vi "Result_Test.vi"(8 "error in (no error)":errorcluster caption="entrée d'erreur (pas d'erreur)", 11 "Get_Voltage en entrée":refnum<class "P2056_Get_SN.lvclass">) -> (0 "error out":errorcluster caption="sortie d'erreur", 3 "Get_Voltage en sortie":refnum<class "P2056_Get_SN.lvclass">)   [LabVIEW 2020, in "Library Test.lvlib" / "P2056_Get_SN.lvclass"]
uses:
  P2056_Get_SN.lvclass
  C:/Users/ngarcin/OneDrive - Altyor/Standard TB/Suite TB45/Class/Test/Test (Default)/Test (Default).lvclass
  Commun VI/TypeDef/Variable Printable.ctl
  JSON API/JSON Value/Set from JSON string.vi
  JSON API/JSON Value/JSON Value.lvclass
  P2056_Send_Command_UART.lvclass
  JSON API/Variant JSON/Variant JSON.lvlib
  JSON API/Get Polymorphic/JSON GetSet.lvlib
  Commun VI/Library Commun.lvlib
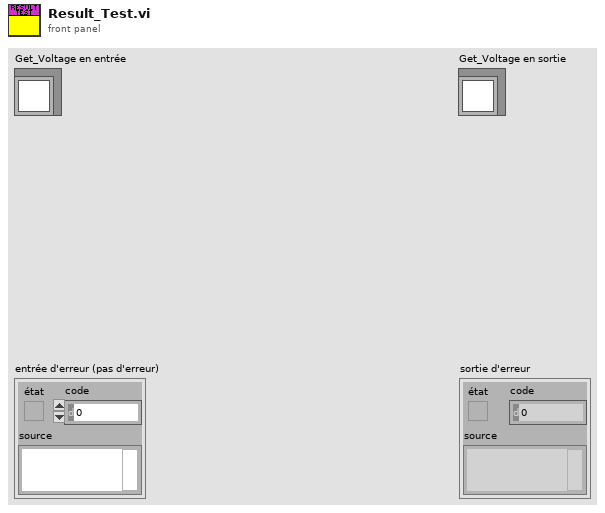
[diagram p1: front panel]
types:
  T1 = typedef "Variable Printable.ctl" = string
  T2 = enum16{"Get Variable", "Get All Variables", "Set Variable", "Delete Variable", "Delete All Variable"}
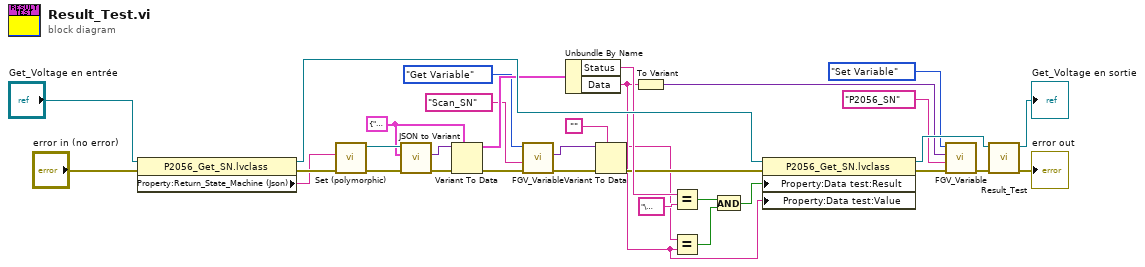
[diagram p0: block diagram]
diagram:
  w26 = cluster{"Data":string, "Status":string} {"Data"="", "Status"=""}
  n1 = property class="P2056_Get_SN.lvclass"(reference="Get_Voltage en entrée", error in="error in (no error)") -> (reference out=w31:refnum<class "P2056_Get_SN.lvclass">, error out=w25:errorcluster, "Property:Return_State_Machine (Json)"=w24:string)
  n2 = call-poly "Set (polymorphic).vi"("error in (no error)"=w25, "JSON stream"=w24) -> ("error out"=w28:errorcluster, "JSON Value out"=w30:refnum<class "JSON Value.lvclass">)  [unwired: 7 in, 1 out]
  n3 = call "JSON to Variant.vi"("error in (no error)"=w28, "Variant (Data Type)"=w26, "JSON Value"=w30) -> ("error out"=w29:errorcluster, "Variant out"=w27:variant)  [unwired: 7 in]
  n4 = Variant To Data(error in=w29, type=w26, Variant=w27) -> (data=w23:cluster{"Data":string, "Status":string}, error out=w9:errorcluster)
  n5 = call "FGV_Variable.vi"("error in (no error)"=w9, "Variable"=T1 "Scan_SN", "Function"=T2."Get Variable") -> ("error out"=w8:errorcluster, "Data Out"=w5:variant)  [unwired: 6 in, 1 out]
  n6 = Unbundle By Name(w23) -> ("Status"=w22:string, "Data"=w4:string)
  n7 = Variant To Data(error in=w8, type="", Variant=w5) -> (data=w3:string, error out=w7:errorcluster)
  n8 = To Variant(anything=w4) -> (Variant=w16:variant)
  n9 = Equal?(x=w22, y="\u0000") -> (x = y?=w20:bool)
  n10 = Equal?(x=w3, y=w4) -> (x = y?=w1:bool)
  n11 = And(x=w20, y=w1) -> (x .and. y?=w2:bool)
  n12 = property class="P2056_Get_SN.lvclass"(reference=w31, error in=w7, "Property:Data test:Result"=w2, "Property:Data test:Value"=w4) -> (reference out=w17:refnum<class "P2056_Get_SN.lvclass">, error out=w13:errorcluster)
  n13 = call "FGV_Variable.vi"("error in (no error)"=w13, "Variable"=T1 "P2056_SN", "Data In"=w16, "Function"=T2."Set Variable") -> ("error out"=w12:errorcluster)  [unwired: 5 in, 2 out]
  n14 = call-parent "Result_Test.vi"("error in (no error)"=w12, "Get_Voltage en entrée"=w17) -> ("error out"=→"error out":errorcluster, "Get_Voltage en sortie"=→"Get_Voltage en sortie":refnum<class "P2056_Get_SN.lvclass">)  [unwired: 8 in]
